vi "i32ToIP (SubVI).vi"(11 "int number":i32) -> (3 "name":string)   [LabVIEW 2017]
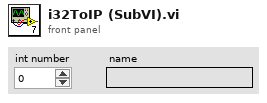
[diagram p1: front panel]
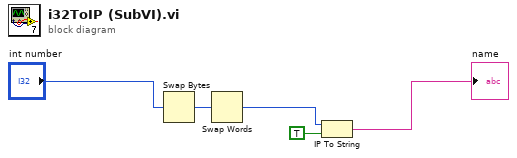
[diagram p0: block diagram]
diagram:
  n1 = Swap Bytes(anything="int number") -> (byte swapped=w1:i32)
  n2 = Swap Words(1:w1) -> (0:w5:i32)
  n3 = IP To String(1:TRUE ("dot notation? (F)"), 2:w5) -> (0:→"name":string)
